vi "LV21_2_2.vi"() -> ()   [LabVIEW 2022 SP3]
panel:
  out "Real Input 2":string="B Y\nA X\nC Z\nA Z\nB Y\nB Y\nA X\nC Z\nB Y\nB Y\nC Z\nC X\nB Y\nC Z\nB Y\nC Z\nA Z\nA Z\nA X\nB Y\nA X\nC Z\nC Y\nC Z\nC Z\nC Z\nA X\nA X\nB Y\nA Z\nB Z\nB Y\nA X\nA X\nC Z\nB Y\nB Y\nB Z\nA Z\nA X\nC Z\nB Z\nA Z\nC Z\nC Z\nC Z\nC Z\nC Z\nC Z\nB X\nA Z\nA Z\nC Z\nC Z\nC Z\nA Y\nC Z\nB Y\nC Z\nC Z\nC Z\nB Y\nB Z\nA X\nA X\nC Z\nB Y\nB Y\nB Z\nA X\nA X\nC Z\nB Y\nC Z\nA X\nC Z\nA X\nC X\nA Y\nA Y\nB Y\nA Y\nC Z\nB Y\nC Z\nC Z\nA X\nC Z\nA Z\nC Z\nA X\nC Z\nB Y\nB Y\nC Z\nB Z\nC Y\nC Z\nB Y\nC Z\nC Z\nB X\nA X\nC Z\nC Z\nB Y\nC Z\nB Y\nA Z\nB Y\nB Z\nA Z\nC Z\nC Z\nC Z\nA Z\nC Z\nA X\nA X\nA Z\nC Z\nA X\nA Z\nC Z\nA Z\nA Y\nB Y\nA Z\nB X\nA X\nC Z\nC Z\nB Y\nC Y\nB Y\nB Z\nB Y\nB Y\nC Z\nC Z\nC Z\nC Z\nA Y\nC Z\nB Z\nA X\nB Y\nA Y\nC Z\nC Z\nC Z\nC Z\nC Z\nB Y\nC Z\nB Y\nC Z\nB Y\nC Z\nC X\nA Y\nA X\nC Y\nB Y\nA Z\nC Z\nC Z\nB Y\nB Y\nA X\nB Y\nA Y\nA X\nA X\nB Y\nA X\nA X\nB Y\nC Z\nC Z\nB Y\nC Z\nA Z\nC Z\nB Z\nC Z\nA Y\nC Z\nB Z\nC Z\nA Y\nA Y\nC Z\nA X\nB Y\nC Z\nA X\nB Y\nB Y\nA X\nA X\nC Z\nB Y\nC Z\nB Z\nC Z\nA X\nC Z\nB Y\nB Y\nA X\nB Z\nC Z\nB Z\nB Y\nB Y\nA Y\nB Z\nA Z\nC Z\nC Z\nA X\nA X\nA X\nC Z\nB Y\nA X\nA Y\nC Z\nA X\nB Y\nA Y\nA Y\nC Z\nC Z\nC Z\nA Z\nB Z\nC Z\nB Y\nC Z\nC Z\nA Y\nA X\nC Z\nB Y\nC Z\nC Z\nB Y\nB Y\nA Y\nC Z\nB Y\nB Y\nA Z\nC Z\nC Z\nC Z\nC Z\nB Z\nC Z\nB Y\nA X\nC Z\nB Z\nA Z\nA X\nC Z\nA X\nA X\nB Y\nC Z\nC Z\nA X\nC Z\nA Y\nC Z\nC Z\nA X\nB Y\nC Z\nB Z\nB Y\nC Z\nA Z\nC Z\nC Z\nA Y\nA Z\nC Z\nC Z\nB Z\nC Z\nB Y\nC Z\nC Z\nA X\nC Z\nC Z\nB Z\nC Z\nB Z\nA X\nB Y\nC Z\nC Z\nC Z\nC Z\nC Z\nA Z\nA Y\nA X\nA X\nC Z\nB X\nA Z\nA X\nC Z\nB Z\nC Z\nB Y\nA Z\nC Z\nB Y\nC Z\nC Y\nA Y\nC Z\nB Y\nB Y\nC Z\nA X\nC Z\nA X\nC X\nA X\nB X\nA X\nC Z\nC Z\nC Z\nB Y\nB Y\nC Z\nB Z\nC Z\nB Y\nA X\nC X\nC Z\nB Y\nA Z\nA X\nB Y\nB Y\nC Z\nC Z\nC Z\nB Y\nA X\nA X\nB Y\nA X\nA Y\nC Z\nB Y\nA X\nA Y\nB Y\nA X\nA X\nC Z\nC Z\nC Z\nC Z\nC Z\nA X\nA X\nB Z\nA Y\nC Z\nA X\nC Z\nB Y\nC Z\nA Z\nC Z\nC Z\nA Y\nB Z\nC Z\nA X\nB Y\nB Y\nC Z\nA Y\nC Z\nC Z\nC Z\nC Z\nC Z\nB Y\nA X\nA X\nB Y\nC Z\nC Z\nA Z\nC Z\nC Z\nC Z\nA Y\nB Z\nB Y\nB Y\nC Z\nA X\nA Y\nC Z\nA X\nA Y\nA X\nC Z\nA Y\nB Z\nB Y\nB Z\nC Z\nC Z\nC Z\nB Z\nB Z\nC Z\nC Z\nC Z\nC Z\nB Y\nB Z\nA Y\nA Y\nB Z\nB X\nA Z\nA X\nC Z\nA X\nA Y\nA X\nA X\nA X\nC Z\nC Z\nC Z\nA X\nC Z\nC Z\nB Y\nA X\nC Z\nA X\nA Y\nA X\nC Z\nA Y\nC Z\nB Y\nA X\nA Y\nA Z\nC Z\nB Y\nB Y\nB Z\nA X\nA X\nB Y\nC Z\nA X\nB Y\nC Z\nC Z\nC Z\nA X\nA Y\nA Z\nC Z\nB Y\nC Z\nA X\nA Z\nA Z\nB Y\nB Y\nA X\nB Y\nC Z\nB Z\nC Z\nB Y\nA Z\nC Z\nA Y\nA X\nA Z\nB Y\nA X\nA Z\nC Z\nA Z\nC Z\nC Z\nA X\nC Z\nA X\nC Z\nA X\nC Z\nB Y\nC Z\nA X\nB Y\nA Y\nC X\nA Y\nA Z\nA X\nA Z\nB Y\nA X\nC Z\nA Y\nB Y\nB Y\nC Z\nB Y\nC Z\nB Y\nB Z\nC Z\nC Z\nB Y\nA X\nC Z\nB Y\nC Z\nC Z\nC Z\nC Z\nC Z\nA X\nA X\nA Z\nA Z\nC Z\nA Y\nB Y\nA Y\nA Y\nB Y\nC X\nA Y\nC Z\nC Z\nC Z\nA Y\nA Y\nA Y\nC Z\nA X\nB Y\nA X\nB X\nA Y\nA Y\nA X\nB Z\nB Y\nC Z\nB Y\nC Z\nB Y\nC Z\nA Z\nC Z\nA X\nB Y\nA X\nC Z\nB Z\nC Z\nB Y\nC Z\nC Z\nC Z\nA X\nA X\nB Y\nB Z\nA Z\nA X\nA X\nC Z\nA X\nA X\nC X\nC X\nC Z\nB Y\nB Z\nC Z\nA X\nB Y\nB Y\nA Z\nC Z\nC Y\nA X\nB Y\nB Y\nC Y\nA X\nA X\nA X\nA X\nA Z\nB Y\nA Z\nC Z\nC Z\nB Y\nB Z\nB Y\nA Y\nC Z\nC Z\nB Y\nA Y\nC Z\nA X\nC Z\nC Z\nA X\nB Y\nC Z\nC Z\nA X\nA Z\nC Z\nA Z\nC Z\nB Z\nA X\nA Y\nB Y\nA X\nA Y\nA Z\nA Y\nA X\nA Y\nC Z\nA X\nC Z\nC Z\nA X\nA Y\nA X\nC Z\nA Z\nC Z\nC Z\nC Z\nA X\nB Y\nA X\nC Z\nC Z\nC Z\nC Z\nA X\nC Z\nC Z\nB Y\nA Y\nA X\nA X\nC Z\nC Z\nA X\nC Z\nC Z\nB Y\nC Z\nA X\nC Z\nC Z\nA Y\nA X\nC Z\nA Y\nC Z\nA X\nB Z\nB Y\nA X\nB Y\nC Z\nA X\nC Z\nC Z\nA X\nC Z\nB X\nC Z\nC Z\nA Y\nC Z\nA Y\nB X\nC Z\nB Y\nC Z\nA Z\nC Z\nA X\nC Z\nC Z\nC Z\nC Z\nA X\nB X\nC Z\nC Z\nB Y\nA Z\nA Y\nC Z\nA X\nA Z\nA X\nA X\nB Y\nA X\nC Z\nA X\nA X\nB Y\nA X\nB Z\nC Z\nA Z\nA Y\nA X\nB Y\nA X\nA Z\nA X\nB Y\nB Z\nB Y\nC Z\nB Y\nA X\nA Y\nC Z\nA X\nB Z\nC Z\nC Z\nA X\nA X\nA Y\nC Z\nC Z\nC Z\nA Y\nB Y\nA X\nC Z\nB Y\nB Y\nA X\nA X\nB Y\nC Z\nB Y\nA X\nA Z\nC Z\nC Z\nC Z\nC Z\nB Z\nC Z\nA Z\nC Z\nA Y\nB Y\nA Y\nC X\nC Z\nC Z\nA Y\nA X\nB Y\nC Z\nA X\nC Z\nA X\nA Y\nA Y\nB Z\nC Y\nB Y\nC Z\nB Y\nA X\nC Z\nC Z\nC Z\nC Z\nB Y\nA X\nB Y\nA Y\nC Z\nB Y\nA Z\nB Z\nC Z\nC Z\nC Z\nC Z\nA Y\nA X\nC Z\nA X\nC Z\nC Z\nC Z\nC Z\nC Z\nB X\nC Z\nB Z\nA X\nA X\nA Y\nA X\nA Z\nB Y\nA Y\nC Z\nC Z\nC Z\nC Z\nC X\nA Y\nC Z\nC Z\nB Y\nA X\nC Y\nB Y\nC Z\nC Z\nC Z\nB X\nA X\nC Z\nA X\nC Z\nC Z\nC Z\nC Y\nA X\nC Z\nA Z\nC Z\nC Z\nB Y\nA X\nA X\nA Z\nA Y\nC Z\nC Z\nC Z\nC Z\nC Z\nC Z\nC Z\nB Y\nA Y\nA X\nC Z\nC Z\nA X\nA X\nC Z\nC Z\nB Y\nA X\nA X\nC Z\nC Z\nC Z\nB Y\nA Y\nB Z\nA Y\nC Z\nA X\nC Z\nC Z\nB Y\nA Y\nA X\nB Z\nA X\nC Z\nC Z\nC Z\nC Z\nB Z\nC Z\nB Y\nC Z\nC Z\nC Z\nB Y\nC Z\nC Y\nB Z\nB Z\nA Y\nC Z\nC Z\nB Z\nB Y\nC Z\nB Y\nC Z\nC Z\nB Y\nC Z\nC Z\nC Z\nA Y\nA X\nB Y\nC Z\nC Z\nC Z\nB Y\nC Z\nA Y\nA X\nA Z\nA Y\nC Z\nC Z\nC Z\nB Z\nC Z\nB Y\nC Z\nB Y\nA Y\nC Z\nC Z\nA Z\nB Y\nA X\nA X\nB Z\nA X\nC Z\nC Z\nC Z\nA X\nB Z\nC Z\nA X\nC Z\nC Z\nC Z\nC Z\nC Z\nC Z\nA Y\nC Z\nA Z\nA X\nB Y\nC Z\nC Z\nA X\nA Y\nC Z\nB Y\nA X\nC Z\nC Z\nA X\nA Y\nA X\nB Z\nC Z\nA X\nC Z\nA X\nA Z\nB Y\nC Z\nC Z\nC X\nB Z\nB X\nB Y\nA Z\nC Z\nA X\nB Z\nA X\nB Y\nC Z\nB Z\nA Z\nA Z\nC Z\nC Z\nC Z\nC Z\nB Y\nB Y\nA Y\nA X\nA X\nB Y\nA Z\nA X\nC Z\nB Z\nA X\nA X\nB Y\nA X\nC Z\nA X\nC Z\nC Z\nC Z\nC Z\nA X\nA X\nA Z\nC Z\nA X\nB Z\nC Z\nB Y\nC Z\nC Z\nA Y\nC Z\nB Z\nC Z\nC Z\nB Y\nC Z\nC Z\nB Y\nA X\nA X\nC Z\nC Z\nC Z\nA X\nC Z\nC Z\nB Y\nC Z\nB Z\nC Z\nA X\nC Z\nA X\nC Z\nA Y\nC Z\nC Z\nA X\nB Y\nC Z\nC Z\nC Z\nA X\nB Y\nC Z\nA X\nB Z\nA X\nB Z\nC Z\nA X\nC Z\nB Y\nA Z\nB X\nA Y\nC Z\nC Z\nB X\nA Y\nA X\nC Z\nA X\nC Z\nB X\nA X\nB Y\nA Z\nA X\nC Z\nA Y\nC Z\nA X\nC Z\nC Z\nC Z\nC Z\nA Z\nC Z\nC Z\nB Y\nA X\nB Y\nC Z\nB Y\nA X\nC Z\nC Z\nA X\nA X\nB Y\nC Z\nB Y\nC Z\nC Z\nA Z\nC Z\nC Z\nC Z\nA Y\nA Z\nC Z\nC Z\nC Z\nC Z\nA X\nC Z\nA X\nA X\nB Z\nC Z\nC Z\nC Z\nB Z\nA X\nC Z\nA Y\nB Y\nC Z\nA Y\nC Z\nC Z\nA X\nA X\nB Y\nA Z\nA Y\nA X\nB X\nB Y\nB Z\nB Y\nA X\nC Z\nC Z\nB Z\nB Z\nB Z\nC Z\nC Z\nB Y\nB Y\nB Y\nC Z\nB Y\nA X\nA Z\nB Z\nA X\nB Z\nA X\nC Z\nB Y\nB X\nA X\nC Z\nA X\nC Z\nC Z\nC Z\nB X\nB Y\nA Y\nA X\nA X\nA Y\nC Z\nC Z\nB Y\nC Z\nB Z\nA X\nC Z\nC Z\nC Z\nA X\nA Y\nC Z\nB Z\nA X\nA Y\nA Z\nC Z\nB Y\nB Z\nA X\nC Z\nA X\nA X\nA Z\nC Z\nC Z\nB Y\nA X\nC Z\nA Y\nA Z\nA X\nA X\nC Z\nA Y\nB Y\nC Z\nA Z\nC Z\nB Y\nA X\nA X\nA X\nC Y\nC Z\nA Y\nB Z\nC X\nA X\nA X\nA X\nA X\nB Z\nB Y\nC Z\nB Y\nA X\nB Y\nC Z\nB Y\nC Z\nC Z\nA X\nB Y\nA Y\nB X\nA X\nB X\nC Z\nA Z\nA X\nB Y\nB Y\nC Z\nA X\nA X\nB Y\nC Z\nA X\nC Z\nA X\nA Z\nA Z\nC Z\nA Z\nC Z\nC Z\nC Z\nC Z\nA Z\nC Y\nC Z\nC Z\nA Z\nA Y\nA X\nB Z\nC Z\nC Z\nC Z\nA Y\nC Z\nC Z\nC Z\nC Z\nA Z\nB Z\nA X\nC Z\nC Z\nA Y\nB Y\nA X\nC Z\nA X\nB Y\nA X\nA X\nA Z\nB Y\nC Z\nB X\nC X\nA X\nA X\nA X\nC Z\nC Z\nA X\nB Y\nA Z\nB Y\nA X\nA Y\nC Z\nB Y\nC Z\nB Y\nA Y\nB Y\nA Y\nA X\nC Z\nC Z\nA X\nB Y\nA X\nC Z\nC Z\nA Y\nB Y\nB Y\nA Z\nB Y\nC Z\nC Z\nC Z\nB Y\nA X\nB Y\nA X\nC Z\nC Z\nC Z\nA X\nC Z\nC Z\nB Y\nC Z\nB Z\nB Y\nA X\nB Y\nA Z\nB Y\nA X\nB X\nC Z\nA Z\nB Y\nC Z\nB Y\nC Z\nC Z\nC Z\nC Z\nB X\nA X\nB Y\nB Y\nA X\nC Z\nA X\nB Z\nB Z\nB Z\nA X\nC X\nA X\nA X\nA X\nB Y\nB Y\nC Z\nC Z\nA X\nC Z\nB Y\nA X\nC Z\nA X\nC Z\nA X\nB Y\nC Z\nC Z\nA Y\nB Y\nC Z\nA Z\nC Z\nA X\nC Z\nC Z\nA Z\nA Y\nC Z\nA X\nB Y\nB Z\nC Z\nA Y\nA Y\nC Z\nC Z\nB Z\nA Z\nC Z\nA X\nC Z\nA X\nC Z\nC Z\nC Z\nB Y\nC Y\nB Y\nA Y\nA X\nC Z\nB Y\nC Z\nC Z\nC Z\nA Z\nC X\nA Y\nC Z\nA Y\nA Y\nC Z\nA Z\nC Z\nC Z\nC Z\nC Z\nC Z\nB Y\nA Y\nB Y\nA Z\nB Y\nA X\nA X\nB Y\nA Z\nB Y\nC Z\nB Z\nA X\nC Z\nA Y\nA Y\nC Z\nA X\nA X\nC Z\nC Z\nC Z\nB Y\nA X\nC Z\nB Y\nC Z\nB X\nC Z\nA Y\nC Z\nA X\nC Z\nA X\nC Z\nC Z\nB Y\nC Z\nB Z\nC Z\nA Y\nA X\nA Z\nC Z\nC Z\nC Z\nC Z\nC Z\nA Z\nB Y\nB Y\nB Y\nC Z\nC Z\nC X\nC Z\nA X\nB Y\nC Z\nC Z\nA X\nB Y\nC Z\nC Z\nC Z\nC Z\nC Z\nC Z\nA X\nB Z\nC Z\nC Z\nC Z\nA X\nB Z\nC Z\nA X\nC Z\nA Y\nB Y\nC Z\nB Z\nB Y\nC Z\nB X\nC Z\nB Y\nB Y\nB Y\nA X\nA X\nC Z\nA Z\nC Z\nB Y\nB Z\nC Z\nC Z\nB Z\nB Y\nA Z\nB Y\nA X\nA X\nC Z\nC Z\nC Z\nB Y\nA X\nC Z\nC Z\nA Y\nC Z\nB Y\nC Z\nC Z\nC Z\nC Z\nC Z\nC Z\nB Y\nB Y\nC Z\nA Z\nA X\nB Y\nC Z\nB Y\nA X\nA Z\nC Z\nB Y\nA Z\nC Z\nB Y\nA Z\nA X\nB Z\nA X\nC Z\nB Y\nC Z\nA Y\nC Y\nA X\nA Y\nC Z\nC Z\nB Y\nC Z\nB Y\nA Z\nC Z\nC Z\nA X\nC Z\nB Z\nA Y\nB Z\nA Z\nA X\nB Y\nA Z\nA Y\nC Z\nC Z\nB Y\nA X\nB Y\nC Z\nA X\nB Y\nB Y\nC Z\nA Z\nA X\nC Z\nB X\nC Z\nC Z\nC Z\nC Y\nA Z\nA X\nC Z\nC Z\nA X\nB Y\nC Z\nB Y\nC Z\nB Z\nA Z\nC Z\nB Y\nA X\nC Z\nC Z\nB Z\nC Z\nA Z\nB Y\nB Z\nC Z\nC Z\nA X\nC Y\nB Y\nC Z\nA X\nC Z\nC Z\nB Y\nB Z\nC Z\nC Z\nA Y\nA X\nC Z\nA X\nB Z\nB Y\nA Z\nB Z\nC X\nA X\nC Z\nC Z\nC Z\nA X\nB Z\nC Z\nC Z\nC Z\nB Y\nC Z\nA X\nC Z\nC Z\nB Y\nC Z\nA X\nC Z\nC Z\nC Z\nA X\nA X\nB Y\nC Z\nC Z\nB Y\nB Z\nB Y\nC Z\nA X\nA X\nB Y\nA X\nB Y\nC Z\nA X\nC Z\nC Z\nB Z\nA X\nB Y\nC Z\nC Z\nC Z\nC Z\nA Z\nC Z\nA X\nB Y\nA Y\nA Y\nC Z\nC Z\nC Z\nB Y\nA Z\nA X\nB Y\nC Z\nA X\nC Z\nA X\nC Z\nA X\nC Z\nC Z\nB Y\nA Y\nC Z\nB Y\nB Y\nA X\nC Z\nA Y\nA Z\nC Z\nC Z\nC Z\nA Y\nB Y\nC Z\nC Z\nB Z\nC Z\nB Z\nB Y\nA X\nA X\nC Z\nB Z\nC Z\nC Z\nA X\nA X\nB Z\nA X\nC Z\nC Z\nB Y\nA X\nC Z\nA X\nB Y\nC X\nA Z\nB Y\nC Z\nA X\nB Y\nC Z\nA X\nB Y\nC Z\nB X\nC Z\nA Y\nC Z\nA X\nC X\nB Z\nC Z\nB Y\nB Y\nB Y\nA Y\nA X\nC Z\nC Z\nA Y\nB Y\nA X\nC Z\nA X\nC Z\nC Z\nA X\nC Z\nA X\nC Z\nB Y\nC Z\nA X\nA Z\nC X\nB Y\nC Z\nC Z\nB Z\nA X\nA X\nB Y\nC Z\nA Y\nB Y\nC Z\nA X\nA Z\nA X\nB Y\nA X\nB Y\nC Z\nC Z\nB Y\nA X\nB Y\nB Z\nC Z\nB Z\nA X\nC Z\nC Z\nA Y\nC Z\nA X\nC Z\nB Y\nC Z\nC Z\nC Y\nC Z\nC Z\nA Y\nC Z\nC Z\nA Z\nA X\nB Z\nC Z\nA Y\nA X\nB Z\nC Z\nC Z\nB Y\nB Z\nA X\nA X\nC Z\nB Y\nA Y\nC Z\nA Z\nA X\nC Z\nA X\nC Z\nC Z\nA Z\nC Z\nC Z\nC Z\nA Y\nB Y\nA X\nB Z\nB Y\nC Z\nC Z\nC Z\nC Z\nC Z\nC Z\nC Z\nA Z\nB Z\nB X\nA X\nA Z\nA X\nA X\nB Y\nC Z\nC Z\nA X\nB Y\nA Y\nC Z\nB Z\nC Z\nA X\nB Y\nC Z\nB Y\nA Z\nC Z\nA Y\nC Z\nA X\nC Z\nA Z\nB Y\nA Y\nA X\nA X\nA Z\nC Z\nC Z\nC Y\nC Z\nA Y\nA X\nB Y\nA Z\nB Z\nB Z\nC Z\nC Z\nC Z\nC Z\nA X\nA Y\nB Y\nC Z\nB Y\nC Z\nA X\nB Y\nC Z\nC Z\nA Z\nA X\nB Y\nC Z\nA Y\nC Z\nC Z\nC Z\nA X\nB Y\nA X\nB Y\nC Z\nC Z\nB Y\nC Z\nA X\nA X\nC Z\nB Y\nB Z\nA X\nA X\nA X\nC Z\nC Z\nB Y\nA X\nC Z\nA X\nA Z\nC Z\nC Z\nC Z\nC Z\nA Z\nA X\nB X\nB Z\nA Y\nC Z\nC Y\nB Y\nC Z\nA Y\nA X\nB Z\nB Y\nC Z\nB Y\nC Z\nA X\nA Z\nA X\nC Z\nB Y\nB Y\nB Y\nA Z\nC Z\nC Z\nB Y\nC Z\nB Y\nA X\nB Y\nA X\nB Y\nC Z\nC Z\nB Y\nA X\nA Y\nB Z\nC Z\nC Z\nA X\nB Y\nA X\nA X\nA Y\nB X\nA X\nA X\nC Z\nB Z\nA X\nC Z\nA Y\nA Z\nC Z\nA Z\nA X\nB Y\nA X\nC X\nC Z\nB Y\nC Z\nA X\nA X\nC Z\nA X\nB Y\nA X\nC Z\nB Z\nC Z\nA X\nC X\nC Z\nC Z\nA X\nC Z\nA Y\nC Z\nA X\nB Y\nB Y\nB Y\nB Y\nB Y\nB Y\nB Y\nB Y\nA Y\nA Z\nB Y\nC Z\nC Z\nB Y\nA Z\nA X\nA Y\nA X\nC Z\nA Y\nA Z\nA Y\nB Y\nC Z\nC Z\nA Y\nC Z\nA X\nB Y\nC Z\nA X\nC Z\nA X\nB Y\nC Z\nC Z\nA Z\nA X\nC Z\nB Y\nA Z\nC Z\nA X\nC Z\nB Y\nB Y\nC Z\nC Z\nC Z\nC Z\nB Z\nC Z\nC Z\nC Z\nC Z\nC Z\nB Y\nB Y\nA X\nC Z\nC Z\nA Z\nC Z\nA X\nC Z\nC Z\nA X\nB Y\nA X\nC Z\nB Y\nB Y\nA Y\nA Y\nA X\nA Y\nA Y\nC Z\nC Z\nA Y\nC Z\nA Y\nB Y\nC Z\nC Z\nC Z\nB Y\nB Y\nB Y\nA X\nC Z\nB Y\nC Z\nC Z\nC Z\nC Z\nA X\nB Y\nA X\nC Z\nA X\nC Y\nA Y\nB Y\nC Z\nC Z\nC Z\nC Z\nB Y\nC Z\nC Z\nB Y\nC Z\nA X\nA X\nB Y\nB X\nC Z\nB Y\nA X\nB Z\nA Z\nC Z\nC Z\nC Z\nC Z\nB Y\nA Z\nC Z\nC Z\nC Z\nC Z\nA X\nA X\nB Y\nA Z\nC Z\nC Z\nC Z\nC Z\nA Z\nB Y\nA X\nB Y\nC Z\nC Z\nB Z\nC Z\nA Y\nC Z\nA Y\nB Y\nC Z\nA X\nC Z\nA X\nB Z\nB Y\nB Y\nA X\nB X\nA X\nC Z\nB Y\nA X\nA Z\nC Z\nC Z\nA Z\nC Z\nC Z\nB Y\nC Y\nC Z\nA Z\nA Z\nC Z\nB X\nC Z\nC Z\nB Y\nC Z\nB Y\nB Y\nA X\nA Y\nB Y\nA X\nB Z\nC Z\nA Z\nA X\nA X\nA Z\nA Z\nB Z\nA X\nB Y\nC Z\nB Y\nA X\nC Z\nB Z\nA Y\nB Z\nC Z\nA X\nB Z\nA X\nA Y\nC Z\nC Z\nC Z\nC Z\nC Z\nA Y\nA Y\nA X\nB Y\nC Z\nA X\nB Y\nA X\nB Y\nC Z\nA Z\nC Z\nC Z\nC Z\nC Z\nC Z\nB Y\nB Z\nC Z\nA X\nA Z\nA X\nA X\nC Z\nC Z\nC Z\nC Z\nB Y\nC Z\nA X\nC Z\nC Z\nC Z\nC Z\nC Z\nB Y\nA Z\nA X\nA Z\nC Z\nC Z\nC Z\nC Z\nB X\nC Z\nC Z\nA X\nC Z\nA Z\nB Z\nB Y\nB Z\nA Y\nB Y\nB Y\nC Z\nA Y\nA Y\nA Y\nC Z\nC Z\nB Z\nA X\nC Z\nA X\nA X\nA X\nC Z\nC Z\nA Z\nA X\nA Y\nC Z\nC Z\nA X\nB Z\nC Z\nA X\nC Z\nA Z\nA X\nC Z\nC Z\nA X\nA Z\nB Y\nA X\nB Y\nC Z\nC Z\nA X\nB Z\nC Z\nB Y\nC Z\nA Z\nC Z\nA X\nB Y\nC Z\nC Z\nA Y\nC X\nA Y\nA Y\nC Z\nC Z\nA X\nA Z\nB Y\nC Z\nB Y\nC Z\nA Y\nC Z\nC Z\nC Z\nA Z\nC Z\nC Z\nB Y\nA Y\nC Z\nC Z\nB Y\nA X\nC Z\nB Y\nC Z\nB Y\nC Z\nB Y\nA X\nA Y\nB Y\nC Z\nB Z\nA Y\nC Z\nA Y\nA Z\nC Z\nB Y\nC Z\nC Z\nB Y\nA Y\nA Y\nC Z\nC Z\nA Y\nC Z\nC X\nC Z\nC Z\nC Z\nA X\nC Z\nB Y\nB Y\nC Z\nC Y\nB Z\nC Z\nB Y\nA X\nA X\nB Y\nC Z\nA X\nC Z\nB Z\nC Z\nA X\nB Y"
  out "Real Input":string
  out "Numeric":i32
  out "Numeric 3":i32
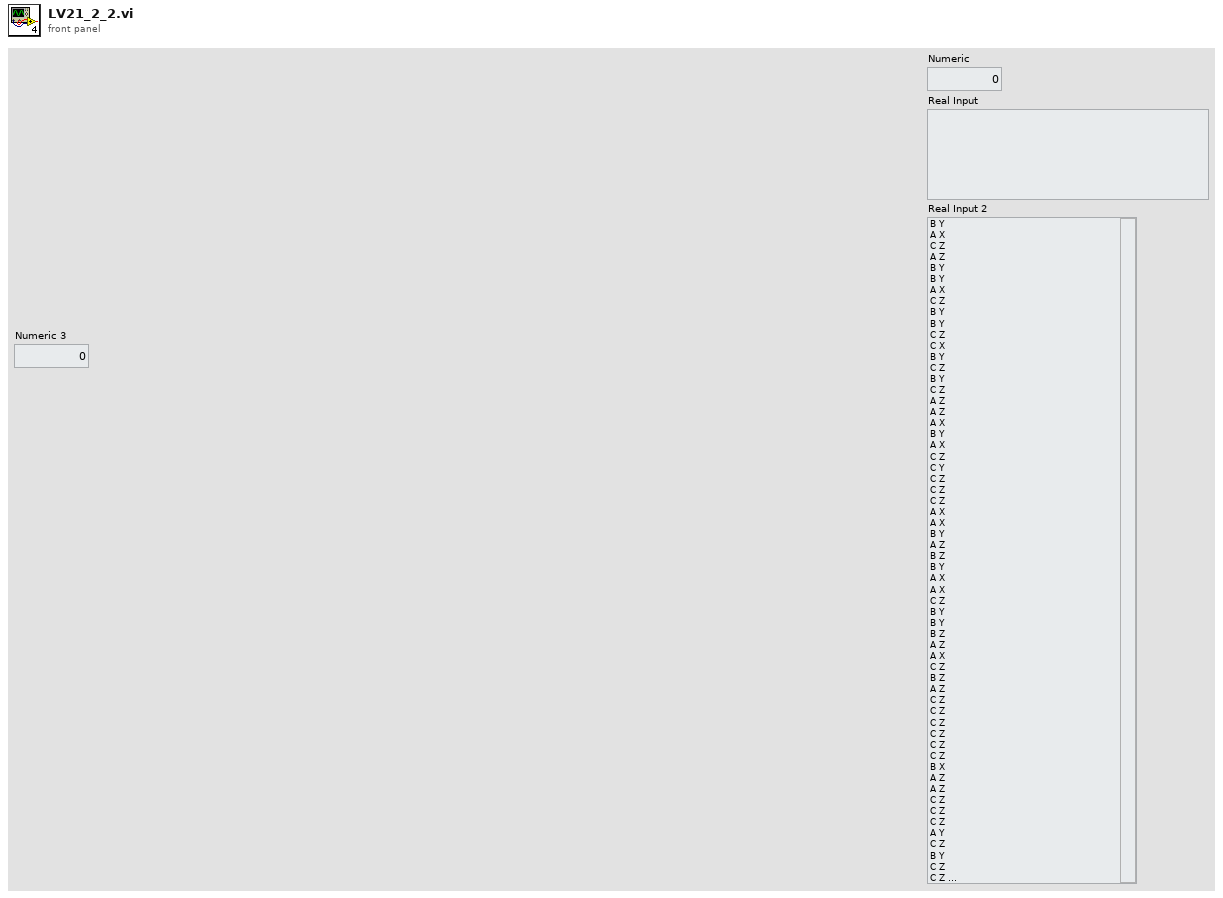
[diagram p1: front panel]
types:
  T1 = enum16{"NOT DEFINED", "Rock", "Paper", "Scissors"}
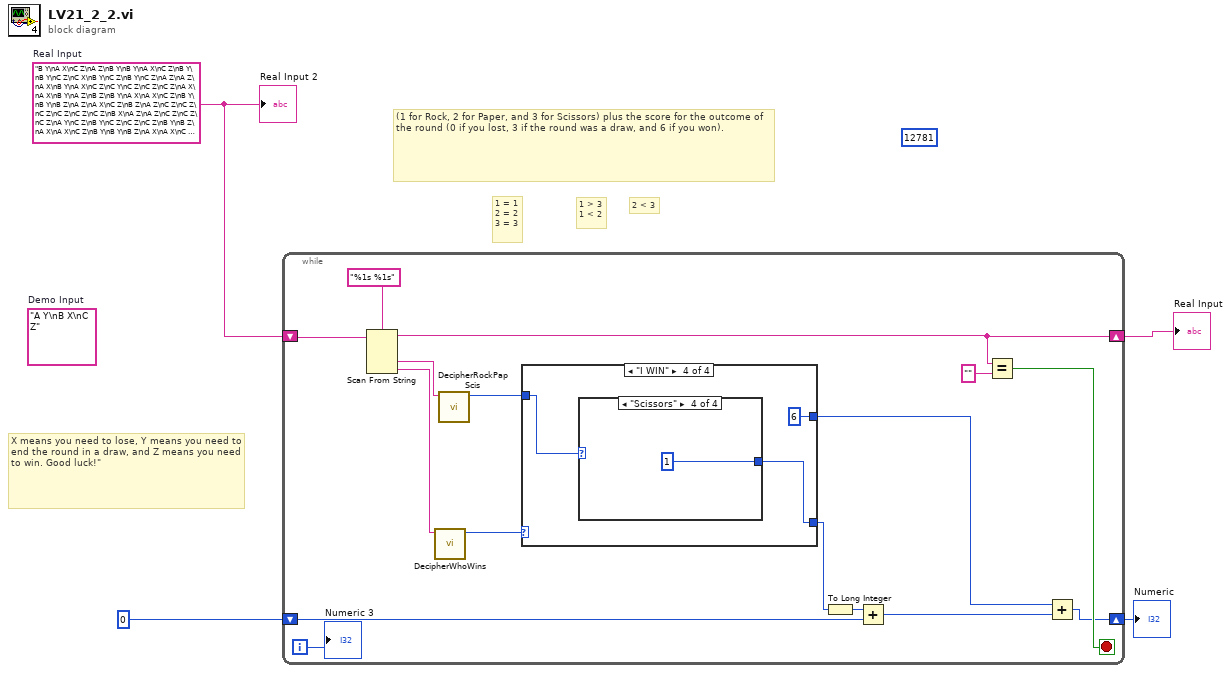
[diagram p0: block diagram]
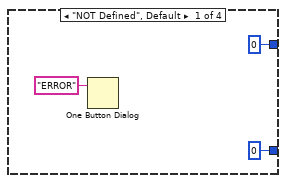
[diagram p2: hidden frame]
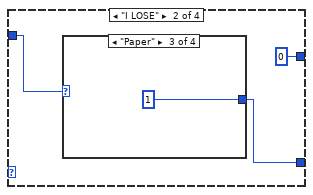
[diagram p3: hidden frame]
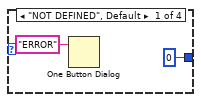
[diagram p4: hidden frame]
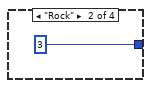
[diagram p5: hidden frame]
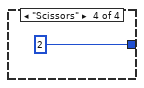
[diagram p6: hidden frame]
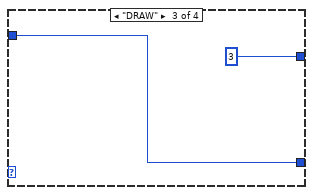
[diagram p7: hidden frame]
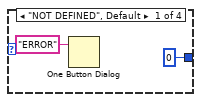
[diagram p8: hidden frame]
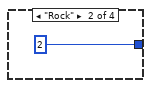
[diagram p9: hidden frame]
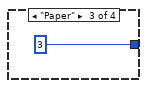
[diagram p10: hidden frame]
diagram:
  (unwired) 12781 ("Numeric 2")
  (unwired) "A Y\nB X\nC Z"  # Demo Input
  w1 = "B Y\nA X\nC Z\nA Z\nB Y\nB Y\nA X\nC Z\nB Y\nB Y\nC Z\nC X\nB Y\nC Z\nB Y\nC Z\nA Z\nA Z\nA X\nB Y\nA X\nC Z\nC Y\nC Z\nC Z\nC Z\nA X\nA X\nB Y\nA Z\nB Z\nB Y\nA X\nA X\nC Z\nB Y\nB Y\nB Z\nA Z\nA X\nC Z\nB Z\nA Z\nC Z\nC Z\nC Z\nC Z\nC Z\nC Z\nB X\nA Z\nA Z\nC Z\nC Z\nC Z\nA Y\nC Z\nB Y\nC Z\nC Z\nC Z\nB Y\nB Z\nA X\nA X\nC Z\nB Y\nB Y\nB Z\nA X\nA X\nC Z\nB Y\nC Z\nA X\nC Z\nA X\nC X\nA Y\nA Y\nB Y\nA Y\nC Z\nB Y\nC Z\nC Z\nA X\nC Z\nA Z\nC Z\nA X\nC Z\nB Y\nB Y\nC Z\nB Z\nC Y\nC Z\nB Y\nC Z\nC Z\nB X\nA X\nC Z\nC Z\nB Y\nC Z\nB Y\nA Z\nB Y\nB Z\nA Z\nC Z\nC Z\nC Z\nA Z\nC Z\nA X\nA X\nA Z\nC Z\nA X\nA Z\nC Z\nA Z\nA Y\nB Y\nA Z\nB X\nA X\nC Z\nC Z\nB Y\nC Y\nB Y\nB Z\nB Y\nB Y\nC Z\nC Z\nC Z\nC Z\nA Y\nC Z\nB Z\nA X\nB Y\nA Y\nC Z\nC Z\nC Z\nC Z\nC Z\nB Y\nC Z\nB Y\nC Z\nB Y\nC Z\nC X\nA Y\nA X\nC Y\nB Y\nA Z\nC Z\nC Z\nB Y\nB Y\nA X\nB Y\nA Y\nA X\nA X\nB Y\nA X\nA X\nB Y\nC Z\nC Z\nB Y\nC Z\nA Z\nC Z\nB Z\nC Z\nA Y\nC Z\nB Z\nC Z\nA Y\nA Y\nC Z\nA X\nB Y\nC Z\nA X\nB Y\nB Y\nA X\nA X\nC Z\nB Y\nC Z\nB Z\nC Z\nA X\nC Z\nB Y\nB Y\nA X\nB Z\nC Z\nB Z\nB Y\nB Y\nA Y\nB Z\nA Z\nC Z\nC Z\nA X\nA X\nA X\nC Z\nB Y\nA X\nA Y\nC Z\nA X\nB Y\nA Y\nA Y\nC Z\nC Z\nC Z\nA Z\nB Z\nC Z\nB Y\nC Z\nC Z\nA Y\nA X\nC Z\nB Y\nC Z\nC Z\nB Y\nB Y\nA Y\nC Z\nB Y\nB Y\nA Z\nC Z\nC Z\nC Z\nC Z\nB Z\nC Z\nB Y\nA X\nC Z\nB Z\nA Z\nA X\nC Z\nA X\nA X\nB Y\nC Z\nC Z\nA X\nC Z\nA Y\nC Z\nC Z\nA X\nB Y\nC Z\nB Z\nB Y\nC Z\nA Z\nC Z\nC Z\nA Y\nA Z\nC Z\nC Z\nB Z\nC Z\nB Y\nC Z\nC Z\nA X\nC Z\nC Z\nB Z\nC Z\nB Z\nA X\nB Y\nC Z\nC Z\nC Z\nC Z\nC Z\nA Z\nA Y\nA X\nA X\nC Z\nB X\nA Z\nA X\nC Z\nB Z\nC Z\nB Y\nA Z\nC Z\nB Y\nC Z\nC Y\nA Y\nC Z\nB Y\nB Y\nC Z\nA X\nC Z\nA X\nC X\nA X\nB X\nA X\nC Z\nC Z\nC Z\nB Y\nB Y\nC Z\nB Z\nC Z\nB Y\nA X\nC X\nC Z\nB Y\nA Z\nA X\nB Y\nB Y\nC Z\nC Z\nC Z\nB Y\nA X\nA X\nB Y\nA X\nA Y\nC Z\nB Y\nA X\nA Y\nB Y\nA X\nA X\nC Z\nC Z\nC Z\nC Z\nC Z\nA X\nA X\nB Z\nA Y\nC Z\nA X\nC Z\nB Y\nC Z\nA Z\nC Z\nC Z\nA Y\nB Z\nC Z\nA X\nB Y\nB Y\nC Z\nA Y\nC Z\nC Z\nC Z\nC Z\nC Z\nB Y\nA X\nA X\nB Y\nC Z\nC Z\nA Z\nC Z\nC Z\nC Z\nA Y\nB Z\nB Y\nB Y\nC Z\nA X\nA Y\nC Z\nA X\nA Y\nA X\nC Z\nA Y\nB Z\nB Y\nB Z\nC Z\nC Z\nC Z\nB Z\nB Z\nC Z\nC Z\nC Z\nC Z\nB Y\nB Z\nA Y\nA Y\nB Z\nB X\nA Z\nA X\nC Z\nA X\nA Y\nA X\nA X\nA X\nC Z\nC Z\nC Z\nA X\nC Z\nC Z\nB Y\nA X\nC Z\nA X\nA Y\nA X\nC Z\nA Y\nC Z\nB Y\nA X\nA Y\nA Z\nC Z\nB Y\nB Y\nB Z\nA X\nA X\nB Y\nC Z\nA X\nB Y\nC Z\nC Z\nC Z\nA X\nA Y\nA Z\nC Z\nB Y\nC Z\nA X\nA Z\nA Z\nB Y\nB Y\nA X\nB Y\nC Z\nB Z\nC Z\nB Y\nA Z\nC Z\nA Y\nA X\nA Z\nB Y\nA X\nA Z\nC Z\nA Z\nC Z\nC Z\nA X\nC Z\nA X\nC Z\nA X\nC Z\nB Y\nC Z\nA X\nB Y\nA Y\nC X\nA Y\nA Z\nA X\nA Z\nB Y\nA X\nC Z\nA Y\nB Y\nB Y\nC Z\nB Y\nC Z\nB Y\nB Z\nC Z\nC Z\nB Y\nA X\nC Z\nB Y\nC Z\nC Z\nC Z\nC Z\nC Z\nA X\nA X\nA Z\nA Z\nC Z\nA Y\nB Y\nA Y\nA Y\nB Y\nC X\nA Y\nC Z\nC Z\nC Z\nA Y\nA Y\nA Y\nC Z\nA X\nB Y\nA X\nB X\nA Y\nA Y\nA X\nB Z\nB Y\nC Z\nB Y\nC Z\nB Y\nC Z\nA Z\nC Z\nA X\nB Y\nA X\nC Z\nB Z\nC Z\nB Y\nC Z\nC Z\nC Z\nA X\nA X\nB Y\nB Z\nA Z\nA X\nA X\nC Z\nA X\nA X\nC X\nC X\nC Z\nB Y\nB Z\nC Z\nA X\nB Y\nB Y\nA Z\nC Z\nC Y\nA X\nB Y\nB Y\nC Y\nA X\nA X\nA X\nA X\nA Z\nB Y\nA Z\nC Z\nC Z\nB Y\nB Z\nB Y\nA Y\nC Z\nC Z\nB Y\nA Y\nC Z\nA X\nC Z\nC Z\nA X\nB Y\nC Z\nC Z\nA X\nA Z\nC Z\nA Z\nC Z\nB Z\nA X\nA Y\nB Y\nA X\nA Y\nA Z\nA Y\nA X\nA Y\nC Z\nA X\nC Z\nC Z\nA X\nA Y\nA X\nC Z\nA Z\nC Z\nC Z\nC Z\nA X\nB Y\nA X\nC Z\nC Z\nC Z\nC Z\nA X\nC Z\nC Z\nB Y\nA Y\nA X\nA X\nC Z\nC Z\nA X\nC Z\nC Z\nB Y\nC Z\nA X\nC Z\nC Z\nA Y\nA X\nC Z\nA Y\nC Z\nA X\nB Z\nB Y\nA X\nB Y\nC Z\nA X\nC Z\nC Z\nA X\nC Z\nB X\nC Z\nC Z\nA Y\nC Z\nA Y\nB X\nC Z\nB Y\nC Z\nA Z\nC Z\nA X\nC Z\nC Z\nC Z\nC Z\nA X\nB X\nC Z\nC Z\nB Y\nA Z\nA Y\nC Z\nA X\nA Z\nA X\nA X\nB Y\nA X\nC Z\nA X\nA X\nB Y\nA X\nB Z\nC Z\nA Z\nA Y\nA X\nB Y\nA X\nA Z\nA X\nB Y\nB Z\nB Y\nC Z\nB Y\nA X\nA Y\nC Z\nA X\nB Z\nC Z\nC Z\nA X\nA X\nA Y\nC Z\nC Z\nC Z\nA Y\nB Y\nA X\nC Z\nB Y\nB Y\nA X\nA X\nB Y\nC Z\nB Y\nA X\nA Z\nC Z\nC Z\nC Z\nC Z\nB Z\nC Z\nA Z\nC Z\nA Y\nB Y\nA Y\nC X\nC Z\nC Z\nA Y\nA X\nB Y\nC Z\nA X\nC Z\nA X\nA Y\nA Y\nB Z\nC Y\nB Y\nC Z\nB Y\nA X\nC Z\nC Z\nC Z\nC Z\nB Y\nA X\nB Y\nA Y\nC Z\nB Y\nA Z\nB Z\nC Z\nC Z\nC Z\nC Z\nA Y\nA X\nC Z\nA X\nC Z\nC Z\nC Z\nC Z\nC Z\nB X\nC Z\nB Z\nA X\nA X\nA Y\nA X\nA Z\nB Y\nA Y\nC Z\nC Z\nC Z\nC Z\nC X\nA Y\nC Z\nC Z\nB Y\nA X\nC Y\nB Y\nC Z\nC Z\nC Z\nB X\nA X\nC Z\nA X\nC Z\nC Z\nC Z\nC Y\nA X\nC Z\nA Z\nC Z\nC Z\nB Y\nA X\nA X\nA Z\nA Y\nC Z\nC Z\nC Z\nC Z\nC Z\nC Z\nC Z\nB Y\nA Y\nA X\nC Z\nC Z\nA X\nA X\nC Z\nC Z\nB Y\nA X\nA X\nC Z\nC Z\nC Z\nB Y\nA Y\nB Z\nA Y\nC Z\nA X\nC Z\nC Z\nB Y\nA Y\nA X\nB Z\nA X\nC Z\nC Z\nC Z\nC Z\nB Z\nC Z\nB Y\nC Z\nC Z\nC Z\nB Y\nC Z\nC Y\nB Z\nB Z\nA Y\nC Z\nC Z\nB Z\nB Y\nC Z\nB Y\nC Z\nC Z\nB Y\nC Z\nC Z\nC Z\nA Y\nA X\nB Y\nC Z\nC Z\nC Z\nB Y\nC Z\nA Y\nA X\nA Z\nA Y\nC Z\nC Z\nC Z\nB Z\nC Z\nB Y\nC Z\nB Y\nA Y\nC Z\nC Z\nA Z\nB Y\nA X\nA X\nB Z\nA X\nC Z\nC Z\nC Z\nA X\nB Z\nC Z\nA X\nC Z\nC Z\nC Z\nC Z\nC Z\nC Z\nA Y\nC Z\nA Z\nA X\nB Y\nC Z\nC Z\nA X\nA Y\nC Z\nB Y\nA X\nC Z\nC Z\nA X\nA Y\nA X\nB Z\nC Z\nA X\nC Z\nA X\nA Z\nB Y\nC Z\nC Z\nC X\nB Z\nB X\nB Y\nA Z\nC Z\nA X\nB Z\nA X\nB Y\nC Z\nB Z\nA Z\nA Z\nC Z\nC Z\nC Z\nC Z\nB Y\nB Y\nA Y\nA X\nA X\nB Y\nA Z\nA X\nC Z\nB Z\nA X\nA X\nB Y\nA X\nC Z\nA X\nC Z\nC Z\nC Z\nC Z\nA X\nA X\nA Z\nC Z\nA X\nB Z\nC Z\nB Y\nC Z\nC Z\nA Y\nC Z\nB Z\nC Z\nC Z\nB Y\nC Z\nC Z\nB Y\nA X\nA X\nC Z\nC Z\nC Z\nA X\nC Z\nC Z\nB Y\nC Z\nB Z\nC Z\nA X\nC Z\nA X\nC Z\nA Y\nC Z\nC Z\nA X\nB Y\nC Z\nC Z\nC Z\nA X\nB Y\nC Z\nA X\nB Z\nA X\nB Z\nC Z\nA X\nC Z\nB Y\nA Z\nB X\nA Y\nC Z\nC Z\nB X\nA Y\nA X\nC Z\nA X\nC Z\nB X\nA X\nB Y\nA Z\nA X\nC Z\nA Y\nC Z\nA X\nC Z\nC Z\nC Z\nC Z\nA Z\nC Z\nC Z\nB Y\nA X\nB Y\nC Z\nB Y\nA X\nC Z\nC Z\nA X\nA X\nB Y\nC Z\nB Y\nC Z\nC Z\nA Z\nC Z\nC Z\nC Z\nA Y\nA Z\nC Z\nC Z\nC Z\nC Z\nA X\nC Z\nA X\nA X\nB Z\nC Z\nC Z\nC Z\nB Z\nA X\nC Z\nA Y\nB Y\nC Z\nA Y\nC Z\nC Z\nA X\nA X\nB Y\nA Z\nA Y\nA X\nB X\nB Y\nB Z\nB Y\nA X\nC Z\nC Z\nB Z\nB Z\nB Z\nC Z\nC Z\nB Y\nB Y\nB Y\nC Z\nB Y\nA X\nA Z\nB Z\nA X\nB Z\nA X\nC Z\nB Y\nB X\nA X\nC Z\nA X\nC Z\nC Z\nC Z\nB X\nB Y\nA Y\nA X\nA X\nA Y\nC Z\nC Z\nB Y\nC Z\nB Z\nA X\nC Z\nC Z\nC Z\nA X\nA Y\nC Z\nB Z\nA X\nA Y\nA Z\nC Z\nB Y\nB Z\nA X\nC Z\nA X\nA X\nA Z\nC Z\nC Z\nB Y\nA X\nC Z\nA Y\nA Z\nA X\nA X\nC Z\nA Y\nB Y\nC Z\nA Z\nC Z\nB Y\nA X\nA X\nA X\nC Y\nC Z\nA Y\nB Z\nC X\nA X\nA X\nA X\nA X\nB Z\nB Y\nC Z\nB Y\nA X\nB Y\nC Z\nB Y\nC Z\nC Z\nA X\nB Y\nA Y\nB X\nA X\nB X\nC Z\nA Z\nA X\nB Y\nB Y\nC Z\nA X\nA X\nB Y\nC Z\nA X\nC Z\nA X\nA Z\nA Z\nC Z\nA Z\nC Z\nC Z\nC Z\nC Z\nA Z\nC Y\nC Z\nC Z\nA Z\nA Y\nA X\nB Z\nC Z\nC Z\nC Z\nA Y\nC Z\nC Z\nC Z\nC Z\nA Z\nB Z\nA X\nC Z\nC Z\nA Y\nB Y\nA X\nC Z\nA X\nB Y\nA X\nA X\nA Z\nB Y\nC Z\nB X\nC X\nA X\nA X\nA X\nC Z\nC Z\nA X\nB Y\nA Z\nB Y\nA X\nA Y\nC Z\nB Y\nC Z\nB Y\nA Y\nB Y\nA Y\nA X\nC Z\nC Z\nA X\nB Y\nA X\nC Z\nC Z\nA Y\nB Y\nB Y\nA Z\nB Y\nC Z\nC Z\nC Z\nB Y\nA X\nB Y\nA X\nC Z\nC Z\nC Z\nA X\nC Z\nC Z\nB Y\nC Z\nB Z\nB Y\nA X\nB Y\nA Z\nB Y\nA X\nB X\nC Z\nA Z\nB Y\nC Z\nB Y\nC Z\nC Z\nC Z\nC Z\nB X\nA X\nB Y\nB Y\nA X\nC Z\nA X\nB Z\nB Z\nB Z\nA X\nC X\nA X\nA X\nA X\nB Y\nB Y\nC Z\nC Z\nA X\nC Z\nB Y\nA X\nC Z\nA X\nC Z\nA X\nB Y\nC Z\nC Z\nA Y\nB Y\nC Z\nA Z\nC Z\nA X\nC Z\nC Z\nA Z\nA Y\nC Z\nA X\nB Y\nB Z\nC Z\nA Y\nA Y\nC Z\nC Z\nB Z\nA Z\nC Z\nA X\nC Z\nA X\nC Z\nC Z\nC Z\nB Y\nC Y\nB Y\nA Y\nA X\nC Z\nB Y\nC Z\nC Z\nC Z\nA Z\nC X\nA Y\nC Z\nA Y\nA Y\nC Z\nA Z\nC Z\nC Z\nC Z\nC Z\nC Z\nB Y\nA Y\nB Y\nA Z\nB Y\nA X\nA X\nB Y\nA Z\nB Y\nC Z\nB Z\nA X\nC Z\nA Y\nA Y\nC Z\nA X\nA X\nC Z\nC Z\nC Z\nB Y\nA X\nC Z\nB Y\nC Z\nB X\nC Z\nA Y\nC Z\nA X\nC Z\nA X\nC Z\nC Z\nB Y\nC Z\nB Z\nC Z\nA Y\nA X\nA Z\nC Z\nC Z\nC Z\nC Z\nC Z\nA Z\nB Y\nB Y\nB Y\nC Z\nC Z\nC X\nC Z\nA X\nB Y\nC Z\nC Z\nA X\nB Y\nC Z\nC Z\nC Z\nC Z\nC Z\nC Z\nA X\nB Z\nC Z\nC Z\nC Z\nA X\nB Z\nC Z\nA X\nC Z\nA Y\nB Y\nC Z\nB Z\nB Y\nC Z\nB X\nC Z\nB Y\nB Y\nB Y\nA X\nA X\nC Z\nA Z\nC Z\nB Y\nB Z\nC Z\nC Z\nB Z\nB Y\nA Z\nB Y\nA X\nA X\nC Z\nC Z\nC Z\nB Y\nA X\nC Z\nC Z\nA Y\nC Z\nB Y\nC Z\nC Z\nC Z\nC Z\nC Z\nC Z\nB Y\nB Y\nC Z\nA Z\nA X\nB Y\nC Z\nB Y\nA X\nA Z\nC Z\nB Y\nA Z\nC Z\nB Y\nA Z\nA X\nB Z\nA X\nC Z\nB Y\nC Z\nA Y\nC Y\nA X\nA Y\nC Z\nC Z\nB Y\nC Z\nB Y\nA Z\nC Z\nC Z\nA X\nC Z\nB Z\nA Y\nB Z\nA Z\nA X\nB Y\nA Z\nA Y\nC Z\nC Z\nB Y\nA X\nB Y\nC Z\nA X\nB Y\nB Y\nC Z\nA Z\nA X\nC Z\nB X\nC Z\nC Z\nC Z\nC Y\nA Z\nA X\nC Z\nC Z\nA X\nB Y\nC Z\nB Y\nC Z\nB Z\nA Z\nC Z\nB Y\nA X\nC Z\nC Z\nB Z\nC Z\nA Z\nB Y\nB Z\nC Z\nC Z\nA X\nC Y\nB Y\nC Z\nA X\nC Z\nC Z\nB Y\nB Z\nC Z\nC Z\nA Y\nA X\nC Z\nA X\nB Z\nB Y\nA Z\nB Z\nC X\nA X\nC Z\nC Z\nC Z\nA X\nB Z\nC Z\nC Z\nC Z\nB Y\nC Z\nA X\nC Z\nC Z\nB Y\nC Z\nA X\nC Z\nC Z\nC Z\nA X\nA X\nB Y\nC Z\nC Z\nB Y\nB Z\nB Y\nC Z\nA X\nA X\nB Y\nA X\nB Y\nC Z\nA X\nC Z\nC Z\nB Z\nA X\nB Y\nC Z\nC Z\nC Z\nC Z\nA Z\nC Z\nA X\nB Y\nA Y\nA Y\nC Z\nC Z\nC Z\nB Y\nA Z\nA X\nB Y\nC Z\nA X\nC Z\nA X\nC Z\nA X\nC Z\nC Z\nB Y\nA Y\nC Z\nB Y\nB Y\nA X\nC Z\nA Y\nA Z\nC Z\nC Z\nC Z\nA Y\nB Y\nC Z\nC Z\nB Z\nC Z\nB Z\nB Y\nA X\nA X\nC Z\nB Z\nC Z\nC Z\nA X\nA X\nB Z\nA X\nC Z\nC Z\nB Y\nA X\nC Z\nA X\nB Y\nC X\nA Z\nB Y\nC Z\nA X\nB Y\nC Z\nA X\nB Y\nC Z\nB X\nC Z\nA Y\nC Z\nA X\nC X\nB Z\nC Z\nB Y\nB Y\nB Y\nA Y\nA X\nC Z\nC Z\nA Y\nB Y\nA X\nC Z\nA X\nC Z\nC Z\nA X\nC Z\nA X\nC Z\nB Y\nC Z\nA X\nA Z\nC X\nB Y\nC Z\nC Z\nB Z\nA X\nA X\nB Y\nC Z\nA Y\nB Y\nC Z\nA X\nA Z\nA X\nB Y\nA X\nB Y\nC Z\nC Z\nB Y\nA X\nB Y\nB Z\nC Z\nB Z\nA X\nC Z\nC Z\nA Y\nC Z\nA X\nC Z\nB Y\nC Z\nC Z\nC Y\nC Z\nC Z\nA Y\nC Z\nC Z\nA Z\nA X\nB Z\nC Z\nA Y\nA X\nB Z\nC Z\nC Z\nB Y\nB Z\nA X\nA X\nC Z\nB Y\nA Y\nC Z\nA Z\nA X\nC Z\nA X\nC Z\nC Z\nA Z\nC Z\nC Z\nC Z\nA Y\nB Y\nA X\nB Z\nB Y\nC Z\nC Z\nC Z\nC Z\nC Z\nC Z\nC Z\nA Z\nB Z\nB X\nA X\nA Z\nA X\nA X\nB Y\nC Z\nC Z\nA X\nB Y\nA Y\nC Z\nB Z\nC Z\nA X\nB Y\nC Z\nB Y\nA Z\nC Z\nA Y\nC Z\nA X\nC Z\nA Z\nB Y\nA Y\nA X\nA X\nA Z\nC Z\nC Z\nC Y\nC Z\nA Y\nA X\nB Y\nA Z\nB Z\nB Z\nC Z\nC Z\nC Z\nC Z\nA X\nA Y\nB Y\nC Z\nB Y\nC Z\nA X\nB Y\nC Z\nC Z\nA Z\nA X\nB Y\nC Z\nA Y\nC Z\nC Z\nC Z\nA X\nB Y\nA X\nB Y\nC Z\nC Z\nB Y\nC Z\nA X\nA X\nC Z\nB Y\nB Z\nA X\nA X\nA X\nC Z\nC Z\nB Y\nA X\nC Z\nA X\nA Z\nC Z\nC Z\nC Z\nC Z\nA Z\nA X\nB X\nB Z\nA Y\nC Z\nC Y\nB Y\nC Z\nA Y\nA X\nB Z\nB Y\nC Z\nB Y\nC Z\nA X\nA Z\nA X\nC Z\nB Y\nB Y\nB Y\nA Z\nC Z\nC Z\nB Y\nC Z\nB Y\nA X\nB Y\nA X\nB Y\nC Z\nC Z\nB Y\nA X\nA Y\nB Z\nC Z\nC Z\nA X\nB Y\nA X\nA X\nA Y\nB X\nA X\nA X\nC Z\nB Z\nA X\nC Z\nA Y\nA Z\nC Z\nA Z\nA X\nB Y\nA X\nC X\nC Z\nB Y\nC Z\nA X\nA X\nC Z\nA X\nB Y\nA X\nC Z\nB Z\nC Z\nA X\nC X\nC Z\nC Z\nA X\nC Z\nA Y\nC Z\nA X\nB Y\nB Y\nB Y\nB Y\nB Y\nB Y\nB Y\nB Y\nA Y\nA Z\nB Y\nC Z\nC Z\nB Y\nA Z\nA X\nA Y\nA X\nC Z\nA Y\nA Z\nA Y\nB Y\nC Z\nC Z\nA Y\nC Z\nA X\nB Y\nC Z\nA X\nC Z\nA X\nB Y\nC Z\nC Z\nA Z\nA X\nC Z\nB Y\nA Z\nC Z\nA X\nC Z\nB Y\nB Y\nC Z\nC Z\nC Z\nC Z\nB Z\nC Z\nC Z\nC Z\nC Z\nC Z\nB Y\nB Y\nA X\nC Z\nC Z\nA Z\nC Z\nA X\nC Z\nC Z\nA X\nB Y\nA X\nC Z\nB Y\nB Y\nA Y\nA Y\nA X\nA Y\nA Y\nC Z\nC Z\nA Y\nC Z\nA Y\nB Y\nC Z\nC Z\nC Z\nB Y\nB Y\nB Y\nA X\nC Z\nB Y\nC Z\nC Z\nC Z\nC Z\nA X\nB Y\nA X\nC Z\nA X\nC Y\nA Y\nB Y\nC Z\nC Z\nC Z\nC Z\nB Y\nC Z\nC Z\nB Y\nC Z\nA X\nA X\nB Y\nB X\nC Z\nB Y\nA X\nB Z\nA Z\nC Z\nC Z\nC Z\nC Z\nB Y\nA Z\nC Z\nC Z\nC Z\nC Z\nA X\nA X\nB Y\nA Z\nC Z\nC Z\nC Z\nC Z\nA Z\nB Y\nA X\nB Y\nC Z\nC Z\nB Z\nC Z\nA Y\nC Z\nA Y\nB Y\nC Z\nA X\nC Z\nA X\nB Z\nB Y\nB Y\nA X\nB X\nA X\nC Z\nB Y\nA X\nA Z\nC Z\nC Z\nA Z\nC Z\nC Z\nB Y\nC Y\nC Z\nA Z\nA Z\nC Z\nB X\nC Z\nC Z\nB Y\nC Z\nB Y\nB Y\nA X\nA Y\nB Y\nA X\nB Z\nC Z\nA Z\nA X\nA X\nA Z\nA Z\nB Z\nA X\nB Y\nC Z\nB Y\nA X\nC Z\nB Z\nA Y\nB Z\nC Z\nA X\nB Z\nA X\nA Y\nC Z\nC Z\nC Z\nC Z\nC Z\nA Y\nA Y\nA X\nB Y\nC Z\nA X\nB Y\nA X\nB Y\nC Z\nA Z\nC Z\nC Z\nC Z\nC Z\nC Z\nB Y\nB Z\nC Z\nA X\nA Z\nA X\nA X\nC Z\nC Z\nC Z\nC Z\nB Y\nC Z\nA X\nC Z\nC Z\nC Z\nC Z\nC Z\nB Y\nA Z\nA X\nA Z\nC Z\nC Z\nC Z\nC Z\nB X\nC Z\nC Z\nA X\nC Z\nA Z\nB Z\nB Y\nB Z\nA Y\nB Y\nB Y\nC Z\nA Y\nA Y\nA Y\nC Z\nC Z\nB Z\nA X\nC Z\nA X\nA X\nA X\nC Z\nC Z\nA Z\nA X\nA Y\nC Z\nC Z\nA X\nB Z\nC Z\nA X\nC Z\nA Z\nA X\nC Z\nC Z\nA X\nA Z\nB Y\nA X\nB Y\nC Z\nC Z\nA X\nB Z\nC Z\nB Y\nC Z\nA Z\nC Z\nA X\nB Y\nC Z\nC Z\nA Y\nC X\nA Y\nA Y\nC Z\nC Z\nA X\nA Z\nB Y\nC Z\nB Y\nC Z\nA Y\nC Z\nC Z\nC Z\nA Z\nC Z\nC Z\nB Y\nA Y\nC Z\nC Z\nB Y\nA X\nC Z\nB Y\nC Z\nB Y\nC Z\nB Y\nA X\nA Y\nB Y\nC Z\nB Z\nA Y\nC Z\nA Y\nA Z\nC Z\nB Y\nC Z\nC Z\nB Y\nA Y\nA Y\nC Z\nC Z\nA Y\nC Z\nC X\nC Z\nC Z\nC Z\nA X\nC Z\nB Y\nB Y\nC Z\nC Y\nB Z\nC Z\nB Y\nA X\nA X\nB Y\nC Z\nA X\nC Z\nB Z\nC Z\nA X\nB Y"  # Real Input
  # "X means you need to lose, Y means you need to end the round in a draw, and Z means you need to win. Good luck!\""
  # "2 < 3"
  # "1 > 3\n1 < 2"
  # "1 = 1\n2 = 2\n3 = 3"
  # "(1 for Rock, 2 for Paper, and 3 for Scissors) plus the score for the outcome of the round (0 if you lost, 3 if the round was a draw, and 6 if you won)."
  n1 = while {
    shift-right: [w18] -> w2
    shift-left: w1 -> [w20]
    shift-right: [w11] -> w3
    shift-left: 0 -> [w13]
    i -> [w10]
    stop <- w16 stop-if-true
    n2 = Scan From String(format string="%1s %1s", input string=w20) -> (remaining string=w18:string, output 1=w15:string, output 2=w9:string)  [unwired: 4 in, 2 out]
    n3 = call "DecipherWhoWins.vi"("A"=w9) -> ("Enum"=w8:enum16{"NOT Defined", "I LOSE", "DRAW", "I WIN"})  [unwired: 10 in]
    n4 = call "DecipherRockPapScis.vi"("A"=w15) -> ("Enum"=w7:T1)  [unwired: 10 in]
    n5 = case shown="\"I WIN\"" w8 {
      tunnel: w7 -> [_ w25 w33 w35]
      tunnel: [0 ("Enum") w24 w33 w34] -> w5
      tunnel: [0 0 3 6] -> w6
      frame "NOT Defined", Default {
        n6 = One Button Dialog(message="ERROR") -> ()  [unwired: 1 in, 1 out]
      }
      frame "I LOSE" {
        n7 = case shown="\"Paper\"" w25 {
          tunnel: [0 3 1 2] -> w24
          frame "NOT DEFINED", Default {
            n8 = One Button Dialog(message="ERROR") -> ()  [unwired: 1 in, 1 out]
          }
          frame "Rock" {
          }
          frame "Paper" {
          }
          frame "Scissors" {
          }
        }
      }
      frame "DRAW" {
      }
      frame "I WIN" {
        n9 = case shown="\"Scissors\"" w35 {
          tunnel: [0 2 3 1] -> w34
          frame "NOT DEFINED", Default {
            n10 = One Button Dialog(message="ERROR") -> ()  [unwired: 1 in, 1 out]
          }
          frame "Rock" {
          }
          frame "Paper" {
          }
          frame "Scissors" {
          }
        }
      }
    }
    n11 = To Long Integer(number=w5) -> (32bit integer=w12:i32)
    n12 = Add(x=w12, y=w13) -> (x+y=w14:i32)
    n13 = Equal?(x=w18, y="") -> (x = y?=w16:bool)
    n14 = Add(x=w6, y=w14) -> (x+y=w11:i32)
    "Numeric 3" <- w10
  }
  "Numeric" <- w3
  "Real Input" <- w2
  "Real Input 2" <- w1
